vi "axex_gui_is_blocked.vi"(1 "error in":errorcluster) -> (0 "gui blocked?":bool)   [LabVIEW 2020, in "AX Excel.lvlib"]
uses:
  AX Excel.lvlib
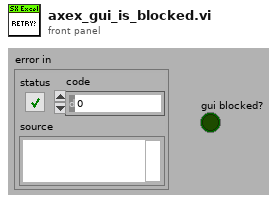
[diagram p1: front panel]
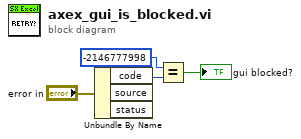
[diagram p0: block diagram]
diagram:
  n1 = Unbundle By Name("error in") -> ("code"=w3:i32)  [unwired: 2 out]
  n2 = Equal?(x=-2146777998, y=w3) -> (x = y?=→"gui blocked?":bool)
